vi "Write Errors to File.vi"(11 "Ground Station Errors":errorcluster) -> (0 "Error Out":errorcluster)   [LabVIEW 2014]
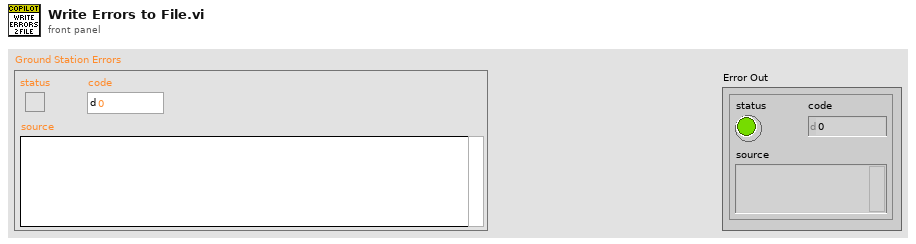
[diagram p1: front panel]
types:
  T1 = cluster{"status":bool, "code":bool, "source":bool}
  T2 = enum16{"open", "replace", "create", "open or create", "replace or create", "replace or create with confirmation"}
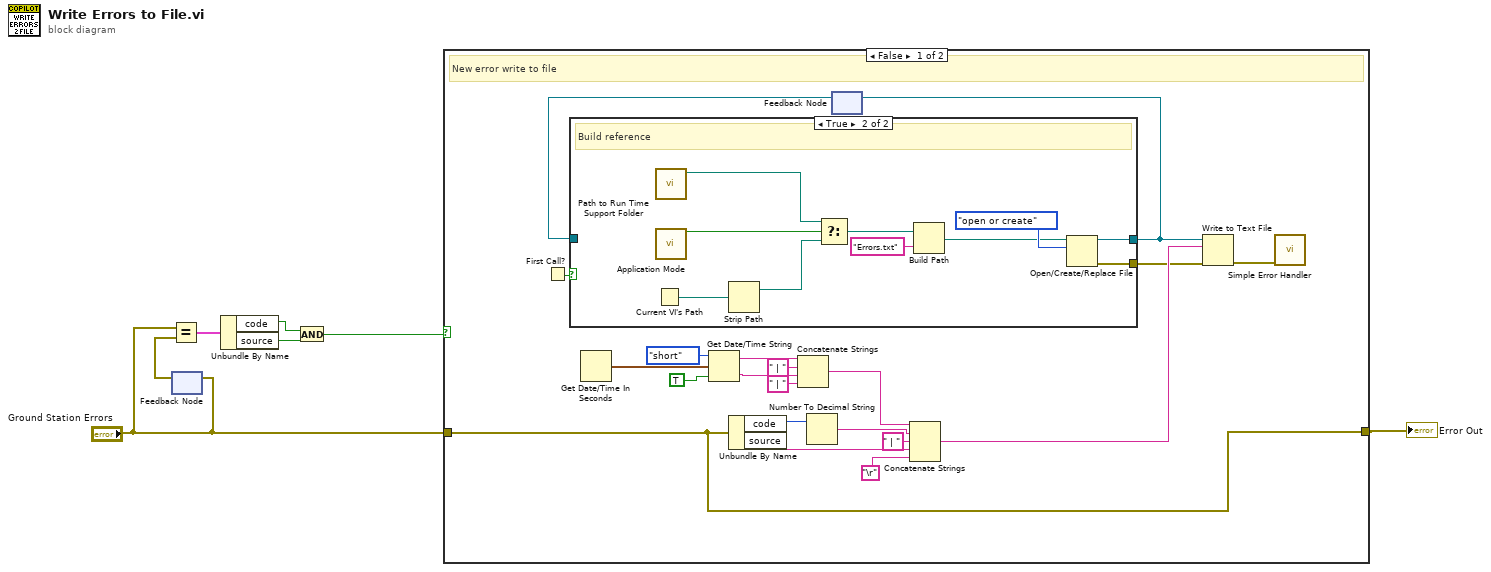
[diagram p0: block diagram]
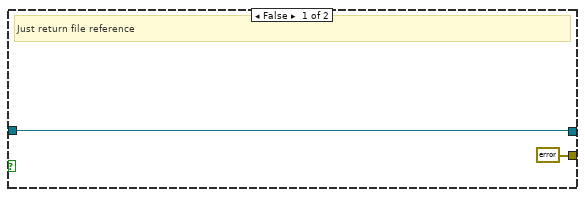
[diagram p2: hidden frame]
diagram:
  n1 = feedback-in #1("Ground Station Errors") -> ()
  n2 = feedback #1() -> (w6:errorcluster)  [unwired: 1 in]
  n3 = Equal?(x="Ground Station Errors", y=w6) -> (x = y?=w5:T1)
  n4 = Unbundle By Name(w5) -> ("code"=w4:bool, "source"=w3:bool)
  n5 = And(x=w4, y=w3) -> (x .and. y?=w2:bool)
  n6 = case shown="False" w2 {
    tunnel: "Ground Station Errors" -> [w8 w40]
    tunnel: [w8 w40] -> w1
    frame False {
      # "New error write to file"
      n7 = First Call?() -> (First Call?: T/F=w13:bool)
      n8 = Get Date/Time In Seconds() -> (seconds since 1Jan1904=w15:timestamp)
      n9 = Get Date/Time String(date format (0)=enum16{"short", "long", "abbreviated"}."short", seconds (now)=w15, want seconds? (F)=TRUE) -> (date string=w22:string, time string=w20:string)
      n10 = Unbundle By Name(w8) -> ("code"=w27:i32, "source"=w24:string)
      n11 = Concatenate Strings(w22, " | " ("string"), w20, " | " ("string")) -> (w18:string)
      n12 = Number To Decimal String(number=w27) -> (decimal integer string=w26:string)  [unwired: 1 in]
      n13 = feedback #2() -> (w11:refnum<file>)  [unwired: 1 in]
      n14 = case shown="True" w13 {
        tunnel: [w29 w33] -> w12
        tunnel: w11 -> [w29 _]
        tunnel: [errorcluster {"status"=FALSE, "code"=0, "source"=""} ("error out") w32] -> w10
        frame False {
          # "Just return file reference"
        }
        frame True {
          # "Build reference"
          n15 = Current VI's Path() -> (path=w31:path)
          n16 = call "Path to Run Time Support Folder.vi"() -> ("Path To Run Time Support Folder"=w38:path)  [unwired: 10 in, 1 out]
          n17 = call "Application Mode.vi"() -> ("Run Time Mode?"=w39:bool)  [unwired: 10 in, 1 out]
          n18 = Strip Path(path=w31) -> (stripped path=w30:path)  [unwired: 1 out]
          n19 = Select(t=w38, s=w39, f=w30) -> (s? t:f=w37:path)
          n20 = Build Path(base path=w37, name or relative path="Errors.txt") -> (appended path=w34:path)
          n21 = Open/Create/Replace File(file path (use dialog)=w34, operation (0:open)=T2."open or create") -> (refnum out=w33:refnum<file>, error out=w32:errorcluster)  [unwired: 4 in, 1 out]
        }
      }
      n22 = feedback-in #2(w12) -> ()
      n23 = Concatenate Strings(w18, w26, " | " ("string"), w24, "\r") -> (w17:string)
      n24 = Write to Text File(file (use dialog)=w12, text=w17, error in=w10) -> (error out=w9:errorcluster)  [unwired: 1 in, 2 out]
      n25 = call <vilib>:"Simple Error Handler.vi"("error in (no error)"=w9) -> ()  [unwired: 4 in, 5 out]
    }
    frame True {
      # "Same error as last time. do not write to file"
    }
  }
  "Error Out" <- w1
